vi "GetThomsonEnable.vi"(11 "Trigger Data":T3) -> (3 "IsThomson":bool)   [LabVIEW 2016]
uses:
  Ctrl_Signal.ctl
  Ctrl_Signal_Map.ctl
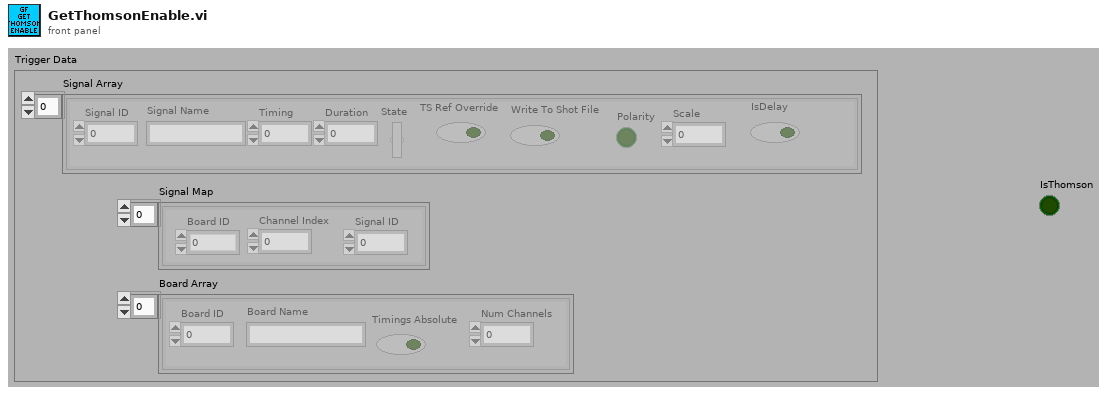
[diagram p1: front panel]
types:
  T1 = typedef "Ctrl_Signal.ctl" = cluster{"Signal Name":string, "Timing":dbl, "Duration":dbl, "State":bool, "TS Ref Override":bool, "Write To Shot File":bool, "Polarity":bool, "Signal ID":dbl, "Scale":dbl, "IsDelay":bool}
  T2 = typedef "Ctrl_Signal_Map.ctl" = cluster{"Channel Index":dbl, "Board ID":dbl, "Signal ID":dbl}
  T3 = cluster{"Signal Array":T1[], "Signal Map":T2[], "Board Array":cluster{"Board ID":dbl, "Board Name":string, "Timings Absolute":bool, "Num Channels":dbl}[]}
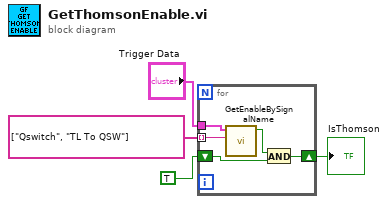
[diagram p0: block diagram]
diagram:
  n1 = for {
    tunnel: string[] ["Qswitch", "TL To QSW"] -> [w9] mode=indexing
    tunnel: "Trigger Data" -> [w8]
    shift-right: [w5] -> w1
    shift-left: TRUE -> [w7]
    n2 = call "GetEnableBySignalName.vi"("Signal Name"=w9, "Trigger Data"=w8) -> ("Signal Enabled"=w6:bool)  [unwired: 9 in]
    n3 = And(x=w6, y=w7) -> (x .and. y?=w5:bool)
  }
  "IsThomson" <- w1
